vi "Close Device.vi"(8 "error in (no error)":errorcluster, 11 "Simulated PSU in":refnum<class "Simulated PSU.lvclass">) -> (0 "error out":errorcluster, 3 "Simulated PSU out":refnum<class "Simulated PSU.lvclass">)   [LabVIEW 2020, in "Simulated PSU.lvlib" / "Simulated PSU.lvclass"]
uses:
  Simulated PSU.lvclass
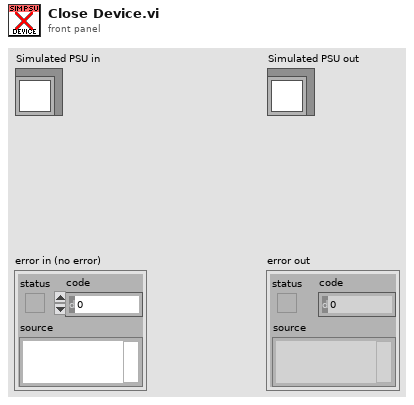
[diagram p1: front panel]
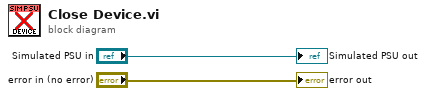
[diagram p0: block diagram]
diagram:
  "error out" <- "error in (no error)"
  "Simulated PSU out" <- "Simulated PSU in"
